vi "Problem1.4.vi"() -> ()   [LabVIEW 2019]
panel:
  out "Edge Change":bool
  out "Edge Off":bool
  out "Edge On":bool
  in  "Boolean\nInput":bool
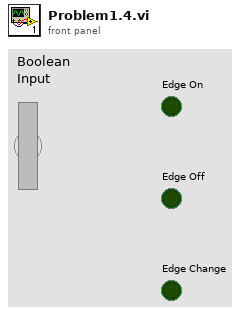
[diagram p1: front panel]
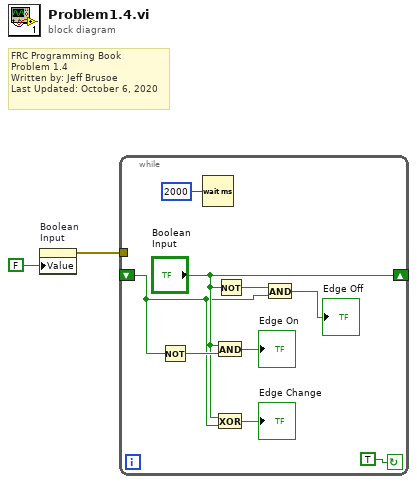
[diagram p0: block diagram]
diagram:
  # "FRC Programming Book\nProblem 1.4\nWritten by: Jeff Brusoe\nLast Updated: October 6, 2020"
  n1 = property on="Boolean\nInput" class="Bool (strict)"("Value"=FALSE ("Boolean\nInput")) -> (error out=w1:errorcluster)  [unwired: 2 in, 1 out]
  n2 = while {
    shift-right: ["Boolean\nInput"] -> _
    shift-left: _ -> [w3]
    tunnel: w1 -> [_]
    stop <- TRUE continue-if-true
    n3 = Not(x=w3) -> (.not. x?=w7:bool)
    n4 = Wait (ms)(milliseconds to wait=u32 2000) -> ()  [unwired: 1 out]
    n5 = And(x="Boolean\nInput", y=w7) -> (x .and. y?=→"Edge On":bool)
    n6 = Exclusive Or(1:w3, 2:"Boolean\nInput") -> (0:→"Edge Change":bool)
    n7 = Not(x="Boolean\nInput") -> (.not. x?=w5:bool)
    n8 = And(x=w5, y=w3) -> (x .and. y?=→"Edge Off":bool)
  }
